vi "Measure PWM Channel.vi"(10 "State":bool, 11 "Settings":T4={"ACTIVE EDGE"=TRUE, "TIMEOUT"=40000000}) -> (3 "Results":T1)   [LabVIEW 2019, in "LRUTS FPGA IP.lvlib" / "Bank.lvclass"]
uses:
  Bank.lvclass
  PWM Acquisition Channel Settings.ctl
  Measure PWM Channel Internal Data.ctl
  PWM Acquisition Channel Measurement.ctl
  PWM Acquisition Channel Results.ctl
  <vilib>/rvi/Emulation/niFpgaSctlEmulationGetInTimedLoop.vi
  <vilib>/rvi/Emulation/niFpgaProcessEmulError.vi
panel:
  out "Measurement":T2
  out "Local.State":bool
  out "Local.Data":T3
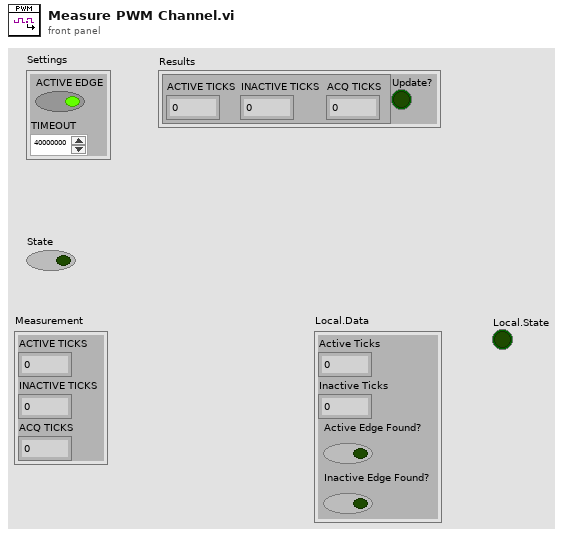
[diagram p1: front panel]
types:
  T1 = typedef "LRUTS FPGA IP.lvlib/Bank.lvclass/PWM Acquisition Channel Results.ctl" = cluster{"Measurement":T2, "Update?":bool}
  T2 = typedef "LRUTS FPGA IP.lvlib/Bank.lvclass/PWM Acquisition Channel Measurement.ctl" = cluster{"ACTIVE TICKS":u32, "INACTIVE TICKS":u32, "ACQ TICKS":u32}
  T3 = typedef "LRUTS FPGA IP.lvlib/Bank.lvclass/Measure PWM Channel Internal Data.ctl" = cluster{"Active Ticks":u32, "Inactive Ticks":u32, "Active Edge Found?":bool, "Inactive Edge Found?":bool}
  T4 = typedef "LRUTS FPGA IP.lvlib/Bank.lvclass/PWM Acquisition Channel Settings.ctl" = cluster{"ACTIVE EDGE":bool, "TIMEOUT":u32}
  T5 = enum8{"Initialize", "Wait on Active Edge", "Wait on Inactive Edge"}
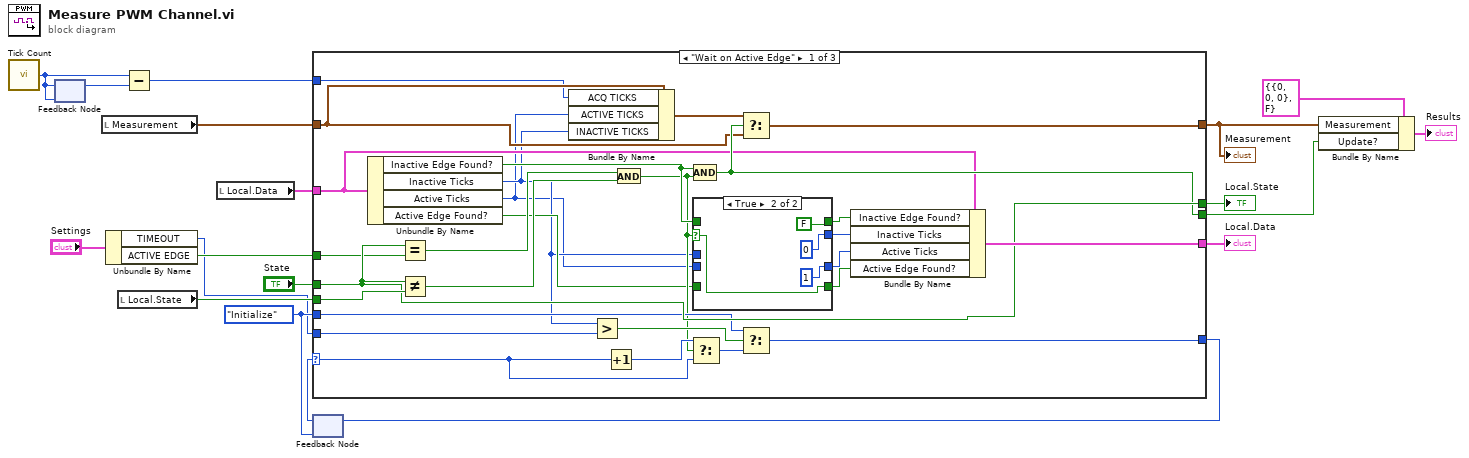
[diagram p0: block diagram]
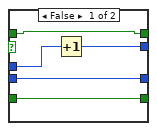
[diagram p2: hidden frame]
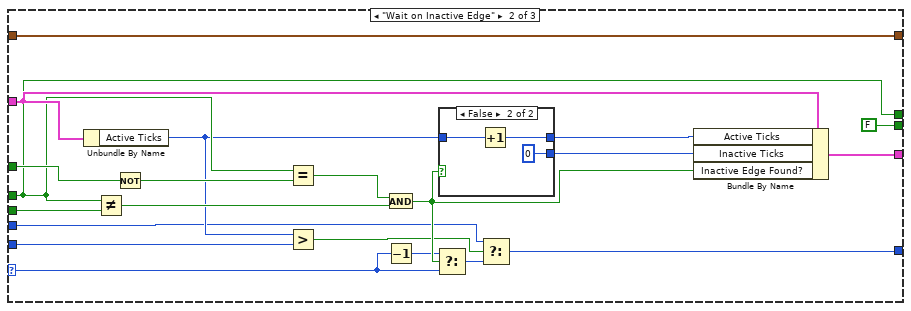
[diagram p3: hidden frame]
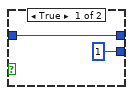
[diagram p4: hidden frame]
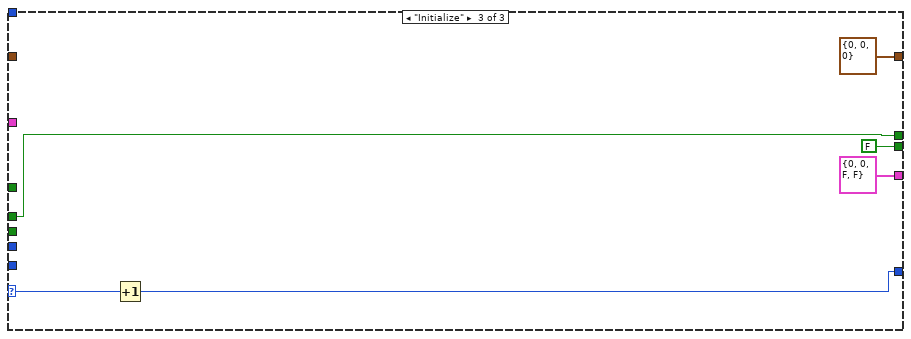
[diagram p5: hidden frame]
diagram:
  w10 = T5."Initialize"
  n1 = call "Tick Count"() -> ("Tick Count(Ticks)"=w7:u32)
  n2 = feedback #1(w7) -> (w8:u32)
  n3 = feedback-in #1(w7) -> ()
  n4 = local read "Measurement"() -> (w12:T2)
  n5 = Unbundle By Name("Settings") -> ("TIMEOUT"=w5:u32, "ACTIVE EDGE"=w15:bool)
  n6 = local read "Local.State"() -> (w13:bool)
  n7 = Subtract(x=w7, y=w8) -> (x-y=w6:u32)
  n8 = local read "Local.Data"() -> (w16:T3)
  n9 = feedback #2(w10) -> (w18:T5)
  n10 = case shown="\"Wait on Active Edge\"" w18 {
    selector: w18 -> [w46 w65 w88]
    tunnel: [w44 w75 T3 {"Active Ticks"=0, "Inactive Ticks"=0, "Active Edge Found?"=FALSE, "Inactive Edge Found?"=FALSE} ("Cached.Data")] -> w19
    tunnel: [w30 w58 w87] -> w17
    tunnel: w16 -> [w25 w74 _]
    tunnel: "State" -> [w39 w67 w86]
    tunnel: w15 -> [w37 w69 _]
    tunnel: [w39 w67 w86] -> w14
    tunnel: w13 -> [w47 w77 _]
    tunnel: [w40 w72 T2 {"ACTIVE TICKS"=0, "INACTIVE TICKS"=0, "ACQ TICKS"=0} ("Cached.Data")] -> w3
    tunnel: w12 -> [w24 w72 _]
    tunnel: w5 -> [w34 w62 _]
    tunnel: w10 -> [w33 w61 _]
    tunnel: [w29 FALSE FALSE] -> w2
    tunnel: w6 -> [w21 _ _]
    frame "Wait on Active Edge" {
      n11 = Unbundle By Name(w25) -> ("Inactive Edge Found?"=w41:bool, "Inactive Ticks"=w22:u32, "Active Ticks"=w20:u32, "Active Edge Found?"=w26:bool)
      n12 = Equal?(x=w39, y=w37) -> (x = y?=w38:bool)
      n13 = Not Equal?(x=w39, y=w47) -> (x != y?=w36:bool)
      n14 = Bundle By Name(cluster=w24, "ACQ TICKS"=w21, "ACTIVE TICKS"=w20, "INACTIVE TICKS"=w22) -> (w23:T2)
      n15 = Greater?(x=w22, y=w34) -> (0:w32:bool)
      n16 = Increment(x=w46) -> (x+1=w45:T5)
      n17 = And(x=w38, y=w36) -> (x .and. y?=w28:bool)
      n18 = Select(t=w45, s=w28, f=w46) -> (s? t:f=w31:T5)
      n19 = case shown="True" w28 {
        selector: w28 -> [_ w53]
        tunnel: [w51 u32 0 ("Inactive time")] -> w43
        tunnel: w22 -> [w52 _]
        tunnel: w41 -> [w50 _]
        tunnel: [w50 FALSE ("Inactive Edge Found?")] -> w42
        tunnel: [w49 u32 1 ("t")] -> w35
        tunnel: w20 -> [w49 _]
        tunnel: [w48 w53] -> w27
        tunnel: w26 -> [w48 _]
        frame False {
          n20 = Increment(x=w52) -> (x+1=w51:u32)
        }
        frame True {
        }
      }
      n21 = Compound Arithmetic op=AND(w41, w28) -> (w29:bool)
      n22 = Select(t=w23, s=w29, f=w24) -> (s? t:f=w40:T2)
      n23 = Select(t=w33, s=w32, f=w31) -> (s? t:f=w30:T5)
      n24 = Bundle By Name(cluster=w25, "Inactive Edge Found?"=w42, "Inactive Ticks"=w43, "Active Ticks"=w35, "Active Edge Found?"=w27) -> (w44:T3)
    }
    frame "Wait on Inactive Edge" {
      n25 = Unbundle By Name(w74) -> ("Active Ticks"=w63:u32)
      n26 = Not Equal?(x=w67, y=w77) -> (x != y?=w76:bool)
      n27 = Not(x=w69) -> (.not. x?=w68:bool)
      n28 = Equal?(x=w67, y=w68) -> (x = y?=w66:bool)
      n29 = Greater?(x=w63, y=w62) -> (0:w60:bool)
      n30 = And(x=w66, y=w76) -> (x .and. y?=w70:bool)
      n31 = Decrement(x=w65) -> (x-1=w64:T5)
      n32 = Select(t=w64, s=w70, f=w65) -> (s? t:f=w59:T5)
      n33 = case shown="False" w70 {
        tunnel: w63 -> [w79 w82]
        tunnel: [w79 w81] -> w73
        tunnel: [u32 1 ("t") u32 0 ("t")] -> w71
        frame True {
        }
        frame False {
          n34 = Increment(x=w82) -> (x+1=w81:u32)
        }
      }
      n35 = Select(t=w61, s=w60, f=w59) -> (s? t:f=w58:T5)
      n36 = Bundle By Name(cluster=w74, "Active Ticks"=w73, "Inactive Ticks"=w71, "Inactive Edge Found?"=w70) -> (w75:T3)
    }
    frame "Initialize" {
      n37 = Increment(x=w88) -> (x+1=w87:T5)
    }
  }
  "Local.Data" <- w19
  "Local.State" <- w14
  "Measurement" <- w3
  n38 = feedback-in #2(w17) -> ()
  n39 = Bundle By Name(cluster=T1 {"Measurement"={"ACTIVE TICKS"=0, "INACTIVE TICKS"=0, "ACQ TICKS"=0}, "Update?"=FALSE} ("PWM Acquisition 0 Results"), "Measurement"=w3, "Update?"=w2) -> (→"Results":T1)
